vi "Setpoint Decision.vi"(11 "input cluster":T1) -> (1 "AI 5 Setpoint":dbl)   [LabVIEW 2011]
uses:
  Robot Global Data.vi
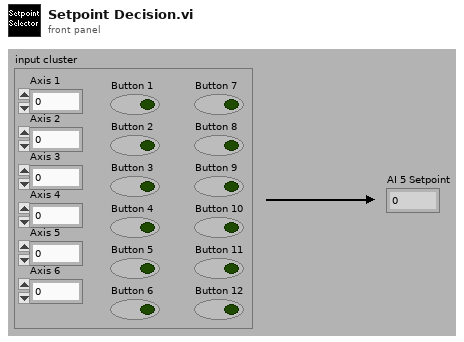
[diagram p1: front panel]
types:
  T1 = cluster{"Axis 1":dbl, "Axis 2":dbl, "Axis 3":dbl, "Axis 4":dbl, "Axis 5":dbl, "Axis 6":dbl, "Button 1":bool, "Button 2":bool, "Button 3":bool, "Button 4":bool, "Button 5":bool, "Button 6":bool, "Button 7":bool, "Button 8":bool, "Button 9":bool, "Button 10":bool, "Button 11":bool, "Button 12":bool}
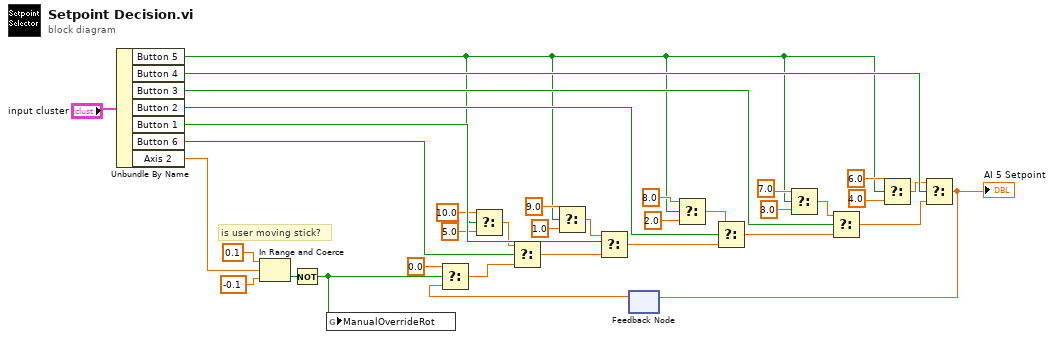
[diagram p0: block diagram]
diagram:
  # "is user moving stick?"
  n1 = Unbundle By Name("input cluster") -> ("Button 5"=w13:bool, "Button 4"=w29:bool, "Button 3"=w30:bool, "Button 2"=w31:bool, "Button 1"=w32:bool, "Button 6"=w1:bool, "Axis 2"=w2:dbl)
  n2 = In Range and Coerce(upper limit=0.1, x=w2, lower limit=-0.1) -> (In Range?=w7:bool)  [unwired: 1 out]
  n3 = Not(x=w7) -> (.not. x?=w3:bool)
  n4 = global write "Robot Global Data.vi" "ManualOverrideRot"(w3) -> ()
  n5 = Select(t=10.0, s=w13, f=5.0) -> (s? t:f=w15:dbl)
  n6 = Select(t=9.0, s=w13, f=1.0 ("t")) -> (s? t:f=w18:dbl)
  n7 = feedback #1() -> (w4:dbl)  [unwired: 1 out]
  n8 = Select(t=0.0, s=w3, f=w4) -> (s? t:f=w9:dbl)
  n9 = Select(t=w15, s=w1, f=w9) -> (s? t:f=w28:dbl)
  n10 = Select(t=w18, s=w32, f=w28) -> (s? t:f=w33:dbl)
  n11 = Select(t=8.0, s=w13, f=2.0 ("t")) -> (s? t:f=w21:dbl)
  n12 = Select(t=w21, s=w31, f=w33) -> (s? t:f=w34:dbl)
  n13 = Select(t=7.0, s=w13, f=3.0 ("t")) -> (s? t:f=w23:dbl)
  n14 = Select(t=w23, s=w30, f=w34) -> (s? t:f=w35:dbl)
  n15 = Select(t=6.0, s=w13, f=4.0 ("t")) -> (s? t:f=w27:dbl)
  n16 = Select(t=w27, s=w29, f=w35) -> (s? t:f=w5:dbl)
  "AI 5 Setpoint" <- w5
  n17 = feedback-in #1(w5) -> ()
